vi "SetTopLeft.vi"(0 "left":i16, 1 "top":i16, 2 "VI Ref":refnum<vi>) -> ()   [LabVIEW 2014]
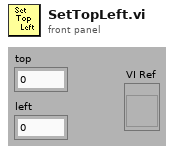
[diagram p1: front panel]
types:
  T1 = typedef "LVRectTypeDef.ctl" = cluster{"Left":i16, "Top":i16, "Right":i16, "Bottom":i16}
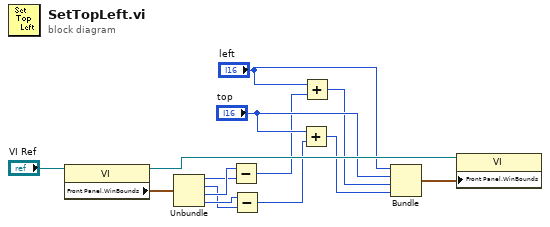
[diagram p0: block diagram]
diagram:
  n1 = property class="VI"(reference="VI Ref") -> (reference out=w8:refnum<vi>, "Front Panel.WinBounds"=w14:T1)  [unwired: 1 in, 1 out]
  n2 = Unbundle(w14) -> ("Left"=w12:i16, "Top"=w10:i16, "Right"=w13:i16, "Bottom"=w11:i16)
  n3 = Subtract(x=w13, y=w12) -> (x-y=w2:i16)
  n4 = Subtract(x=w11, y=w10) -> (x-y=w1:i16)
  n5 = Add(x="top", y=w1) -> (x+y=w3:i16)
  n6 = Add(x="left", y=w2) -> (x+y=w4:i16)
  n7 = Bundle("left"="left", "top"="top", w4, w3) -> (w5:cluster{"left":i16, "top":i16, i16, i16})  [unwired: 1 in]
  n8 = property class="VI"(reference=w8, "Front Panel.WinBounds"=w5) -> ()  [unwired: 1 in, 2 out]
